vi "Load_Position_Limit.vi"(0 "Serial In":refnum<visa-resource-name>, 5 "Node":i32, 7 "Upper Limit":i64, 9 "Lower Limit":i64, 11 "Error In":errorcluster) -> (4 "Serial Out":refnum<visa-resource-name>, 15 "Error Out":errorcluster)   [LabVIEW 2018]
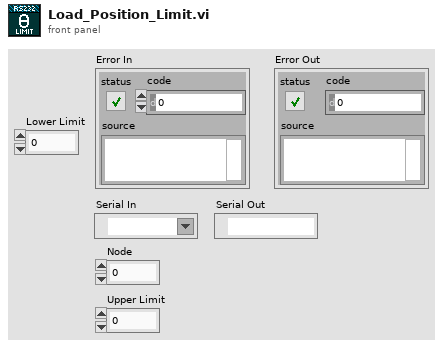
[diagram p1: front panel]
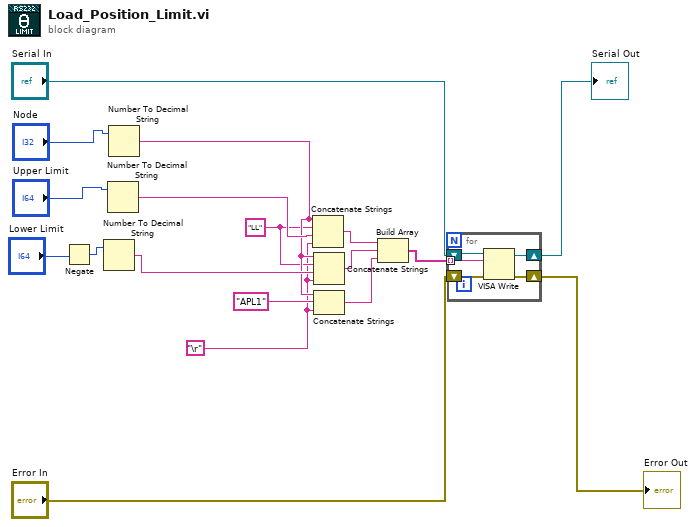
[diagram p0: block diagram]
diagram:
  w7 = "LL" ("string")
  w5 = "\r"
  n1 = Negate(x="Lower Limit") -> (-x=w10:i64)
  n2 = Number To Decimal String(number=w10) -> (decimal integer string=w9:string)  [unwired: 1 in]
  n3 = Number To Decimal String(number="Upper Limit") -> (decimal integer string=w12:string)  [unwired: 1 in]
  n4 = Number To Decimal String(number="Node") -> (decimal integer string=w8:string)  [unwired: 1 in]
  n5 = Concatenate Strings(w8, w7, w12, w5) -> (w4:string)
  n6 = Concatenate Strings(w8, w7, w9, w5) -> (w3:string)
  n7 = Concatenate Strings(w8, "APL1" ("string"), w5) -> (w2:string)
  n8 = Build Array(w4, w3, w2) -> (w1:string[])
  n9 = for {
    tunnel: w1 -> [w19] mode=indexing
    shift-right: [w20] -> w15
    shift-left: "Serial In" -> [w23]
    shift-right: [w21] -> w16
    shift-left: "Error In" -> [w22]
    n10 = VISA Write(VISA resource name=w23, write buffer=w19, error in (no error)=w22) -> (VISA resource name out=w20:refnum<visa-resource-name>, error out=w21:errorcluster)  [unwired: 1 out]
  }
  "Error Out" <- w16
  "Serial Out" <- w15
